vi "Configure Frequency Response Analysis.vi"(0 "VISA resource name":refnum<visa-resource-name>, 1 "Input Source (0: Channel 1)":i32(ring) items=["Channel 1", "Channel 2", "Channel 3", "Channel 4"], 2 "Input Voltage Amplitude (1 Volts)":dbl=1.0, 5 "Stop Frequency (0: 100Hz)":i32(ring) items=["100Hz", "1KHz", "10KHz", "100KHz", "1MHz", "10MHz", "20MHz"], 7 "Start Frequency (0: 20Hz)":i32(ring) items=["20Hz", "100Hz", "1KHz", "10KHz", "100KHz", "1MHz", "10MHz", "10Hz", "20MHz"], 9 "Enable Frequency Response Analysis (F: Disable)":bool, 11 "error in (no error)":errorcluster, 12 "Output Source (1: Channel 2)":i32(ring)=1 items=["Channel 1", "Channel 2", "Channel 3", "Channel 4"], 13 "Load Resistance (0: 1 Mohm)":i32(ring) items=["1 Mohm", "50 ohm"]) -> (4 "VISA resource name out":refnum<visa-resource-name>, 15 "error out":errorcluster)   [LabVIEW 2015, in "Agilent 2000 3000 X-Series.lvlib"]
doc: "Configures frequency response analysis."
uses:
  Agilent 2000 3000 X-Series.lvlib
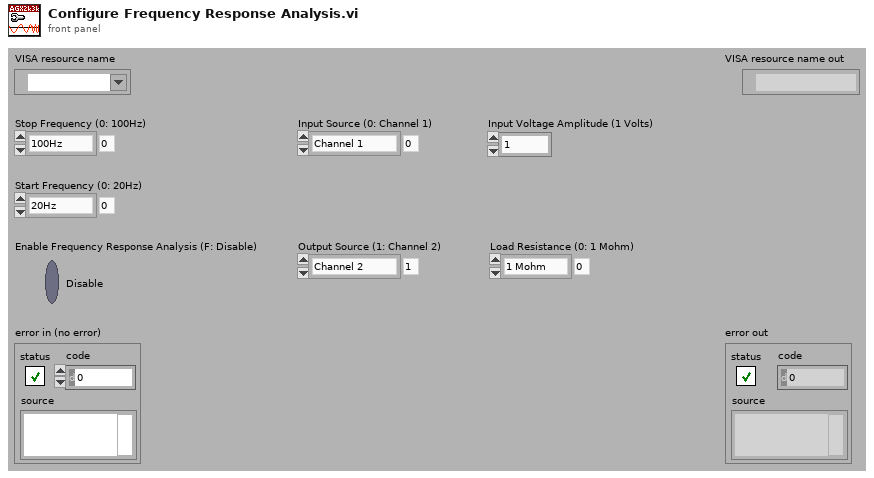
[diagram p1: front panel]
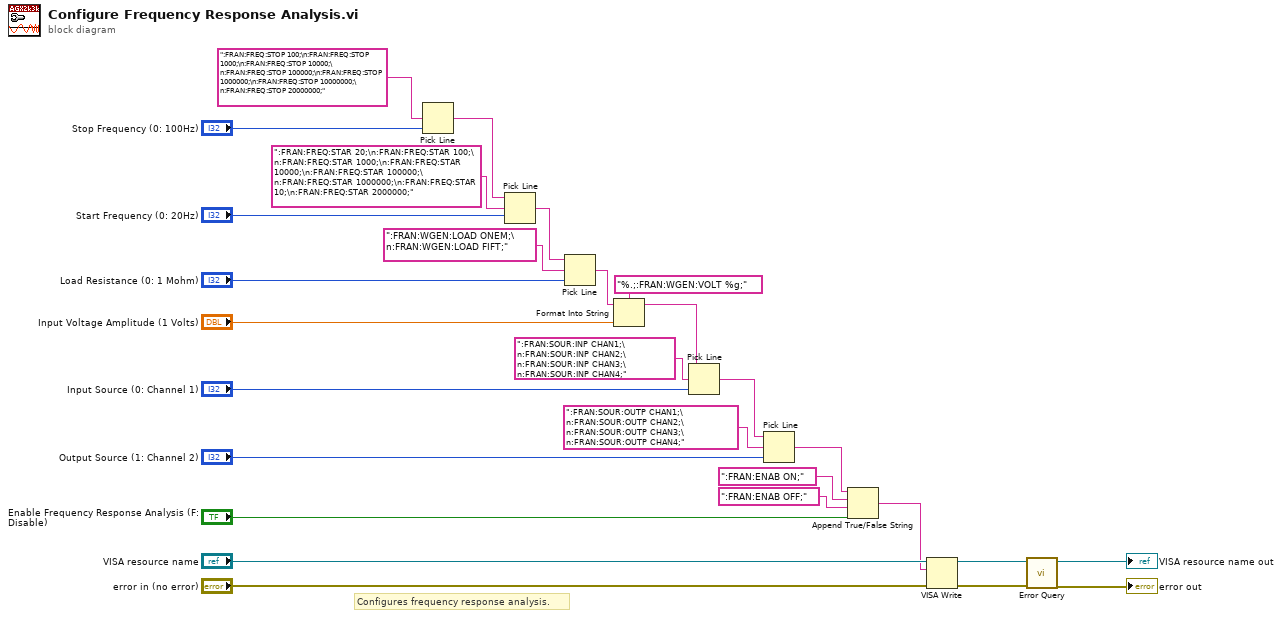
[diagram p0: block diagram]
diagram:
  # "Configures frequency response analysis."
  n1 = Pick Line(multi-line string=":FRAN:FREQ:STOP 100;\n:FRAN:FREQ:STOP 1000;\n:FRAN:FREQ:STOP 10000;\n:FRAN:FREQ:STOP 100000;\n:FRAN:FREQ:STOP 1000000;\n:FRAN:FREQ:STOP 10000000;\n:FRAN:FREQ:STOP 20000000;", line index="Stop Frequency (0: 100Hz)") -> (output string=w3:string)  [unwired: 1 in]
  n2 = Pick Line(string ("")=w3, multi-line string=":FRAN:FREQ:STAR 20;\n:FRAN:FREQ:STAR 100;\n:FRAN:FREQ:STAR 1000;\n:FRAN:FREQ:STAR 10000;\n:FRAN:FREQ:STAR 100000;\n:FRAN:FREQ:STAR 1000000;\n:FRAN:FREQ:STAR 10;\n:FRAN:FREQ:STAR 2000000;", line index="Start Frequency (0: 20Hz)") -> (output string=w2:string)
  n3 = Pick Line(string ("")=w2, multi-line string=":FRAN:WGEN:LOAD ONEM;\n:FRAN:WGEN:LOAD FIFT;", line index="Load Resistance (0: 1 Mohm)") -> (output string=w23:string)
  n4 = Format Into String(format string="%.;:FRAN:WGEN:VOLT %g;", initial string=w23, "Input Voltage Amplitude (1 Volts)") -> (resulting string=w18:string)  [unwired: 1 in, 1 out]
  n5 = Pick Line(string ("")=w18, multi-line string=":FRAN:SOUR:INP CHAN1;\n:FRAN:SOUR:INP CHAN2;\n:FRAN:SOUR:INP CHAN3;\n:FRAN:SOUR:INP CHAN4;", line index="Input Source (0: Channel 1)") -> (output string=w15:string)
  n6 = Pick Line(string ("")=w15, multi-line string=":FRAN:SOUR:OUTP CHAN1;\n:FRAN:SOUR:OUTP CHAN2;\n:FRAN:SOUR:OUTP CHAN3;\n:FRAN:SOUR:OUTP CHAN4;", line index="Output Source (1: Channel 2)") -> (output string=w8:string)
  n7 = Append True/False String(1:"Enable Frequency Response Analysis (F: Disable)", 2:":FRAN:ENAB OFF;", 3:":FRAN:ENAB ON;", 4:w8) -> (0:w7:string)
  n8 = VISA Write(VISA resource name="VISA resource name", write buffer=w7, error in (no error)="error in (no error)") -> (VISA resource name out=w12:refnum<visa-resource-name>, error out=w11:errorcluster)  [unwired: 1 out]
  n9 = call "Error Query.vi"("error in (no error)"=w11, "VISA resource name"=w12) -> ("error out"=→"error out":errorcluster, "VISA resource name out"=→"VISA resource name out":refnum<visa-resource-name>)  [unwired: 6 in, 2 out]
